vi "Configure Spurious Emission (Segment Sweep And Trace Setup).vi"(0 "VISA resource name":refnum<visa-resource-name>, 1 "Spurious Detection Mode":i32[](array[ring]) items=["Normal", "Positive", "Sample", "Negative", "RMS"], 5 "Spurious Mode (1:On)":i32(ring)=1 items=["Off", "On"], 7 "Spurious Auto Sweep Time":i32[](array[ring]) items=["Auto", "Manual"], 9 "Spurious Trace Point":i32[](array[ring]) items=["11", "21", "41", "51", "101", "201", "251", "401", "501", "1001", "2001", "5001", "10001"], 11 "error in (no error)":errorcluster, 12 "Spurious Storage Count":i32[](array[numeric]) min=2 max=9999, 13 "Spurious Sweep Time":dbl[](array[numeric]) min=0.001 max=1000.0) -> (4 "VISA resource name out":refnum<visa-resource-name>, 15 "error out":errorcluster)   [LabVIEW 2020, in "Anritsu Signal Analyzer Series.lvlib"]
doc: "Configures the sweep and trace for segment parameter of Spurious Emission measurement."
uses:
  Anritsu Signal Analyzer Series.lvlib
panel:
  # "s"
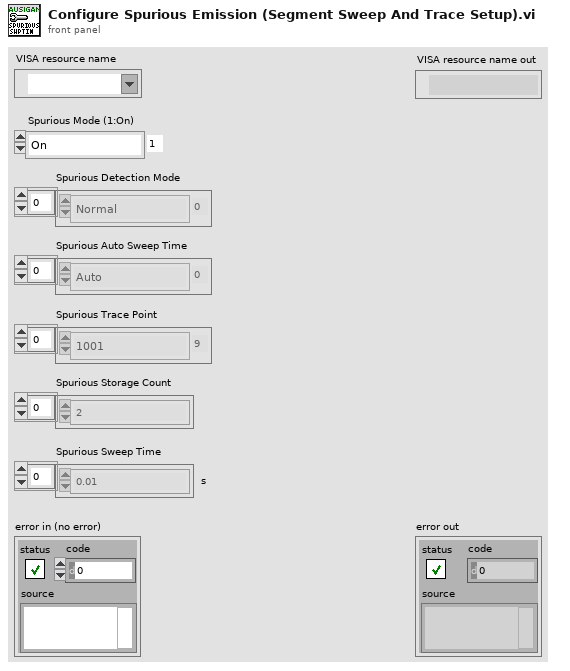
[diagram p1: front panel]
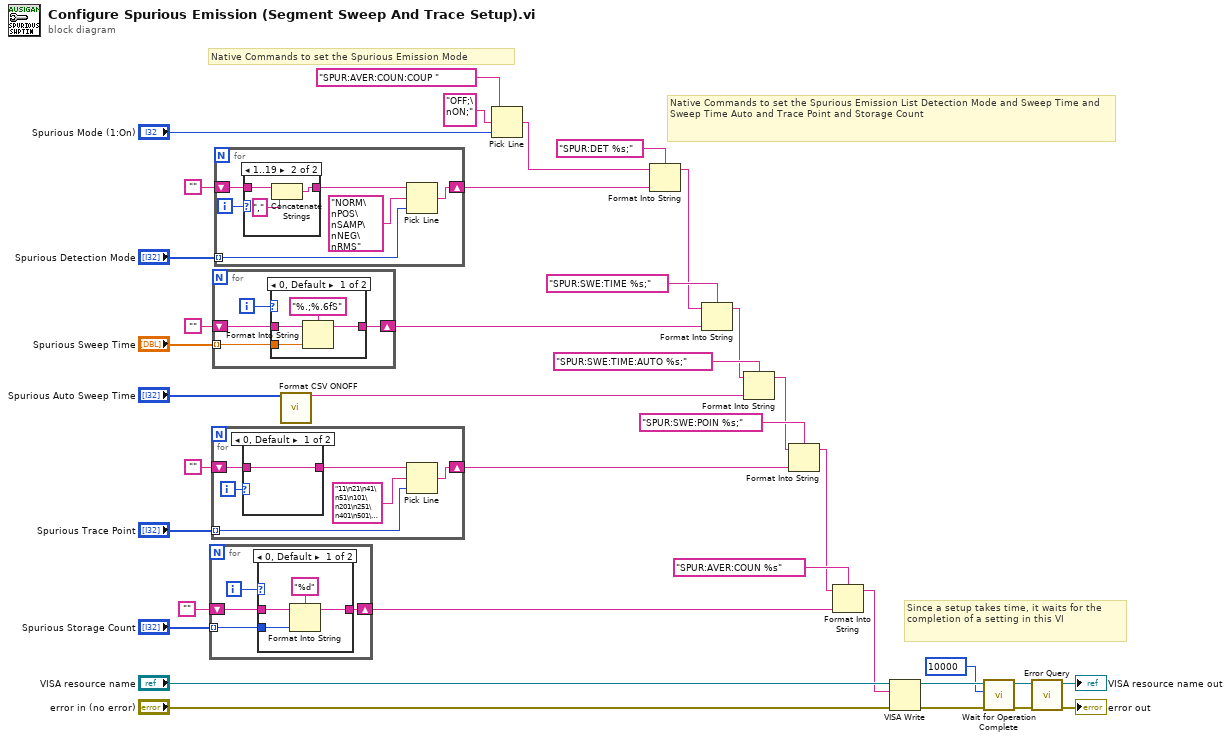
[diagram p0: block diagram]
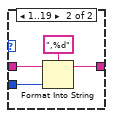
[diagram p2: hidden frame]
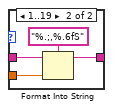
[diagram p3: hidden frame]
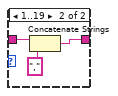
[diagram p4: hidden frame]
diagram:
  # "Since a setup takes time, it waits for the completion of a setting in this VI"
  # "Native Commands to set the Spurious Emission List Detection Mode and Sweep Time and Sweep Time Auto and Trace Point and Storage Count"
  # "Native Commands to set the Spurious Emission Mode"
  n1 = for {
    shift-right: [w38] -> w14
    shift-left: "" -> [w40]
    tunnel: "Spurious Storage Count" -> [w39] mode=indexing
    i -> [w41]
    n2 = case shown="0, Default" w41 {
      tunnel: w40 -> [w44 w47]
      tunnel: [w42 w46] -> w38
      tunnel: w39 -> [w43 w48]
      frame 0, Default {
        n3 = Format Into String(format string="%d" ("string"), initial string=w44, w43) -> (resulting string=w42:string)  [unwired: 1 in, 1 out]
      }
      frame 1..19 {
        n4 = Format Into String(format string=",%d" ("string"), initial string=w47, w48) -> (resulting string=w46:string)  [unwired: 1 in, 1 out]
      }
    }
  }
  n5 = for {
    shift-right: [w50] -> w22
    shift-left: "" -> [w54]
    tunnel: "Spurious Trace Point" -> [w51] mode=indexing
    i -> [w55]
    n6 = case shown="0, Default" w55 {
      tunnel: w54 -> [w56 w59]
      tunnel: [w56 w57] -> w52
      frame 0, Default {
      }
      frame 1..19 {
        n7 = Concatenate Strings(w59, "," ("string")) -> (w57:string)
      }
    }
    n8 = Pick Line(string ("")=w52, multi-line string="11\n21\n41\n51\n101\n201\n251\n401\n501\n1001\n2001\n5001\n10001" ("複数行文字列"), line index=w51) -> (output string=w50:string)
  }
  n9 = for {
    shift-right: [w60] -> w16
    shift-left: "" -> [w62]
    tunnel: "Spurious Sweep Time" -> [w61] mode=indexing
    i -> [w63]
    n10 = case shown="0, Default" w63 {
      tunnel: w62 -> [w66 w69]
      tunnel: [w64 w68] -> w60
      tunnel: w61 -> [w65 w70]
      frame 0, Default {
        n11 = Format Into String(format string="%.;%.6fS" ("string"), initial string=w66, w65) -> (resulting string=w64:string)  [unwired: 1 in, 1 out]
      }
      frame 1..19 {
        n12 = Format Into String(format string="%.;,%.6fS" ("string"), initial string=w69, w70) -> (resulting string=w68:string)  [unwired: 1 in, 1 out]
      }
    }
  }
  n13 = for {
    shift-right: [w73] -> w27
    shift-left: "" -> [w76]
    tunnel: "Spurious Detection Mode" -> [w72] mode=indexing
    i -> [w77]
    n14 = case shown="1..19" w77 {
      tunnel: w76 -> [w78 w81]
      tunnel: [w78 w79] -> w74
      frame 0, Default {
      }
      frame 1..19 {
        n15 = Concatenate Strings(w81, "," ("string")) -> (w79:string)
      }
    }
    n16 = Pick Line(string ("")=w74, multi-line string="NORM\nPOS\nSAMP\nNEG\nRMS" ("複数行文字列"), line index=w72) -> (output string=w73:string)
  }
  n17 = call "Format CSV ONOFF.vi"("Data_In"="Spurious Auto Sweep Time") -> ("Data_out"=w4:string)  [unwired: 14 in]
  n18 = Pick Line(string ("")="SPUR:AVER:COUN:COUP " ("_CommandSet"), multi-line string="OFF;\nON;" ("複数行文字列"), line index="Spurious Mode (1:On)") -> (output string=w8:string)
  n19 = Format Into String(format string="SPUR:DET %s;" ("_CommandSet"), initial string=w8, w27) -> (resulting string=w13:string)  [unwired: 1 in, 1 out]
  n20 = Format Into String(format string="SPUR:SWE:TIME %s;" ("_CommandSet"), initial string=w13, w16) -> (resulting string=w12:string)  [unwired: 1 in, 1 out]
  n21 = Format Into String(format string="SPUR:SWE:TIME:AUTO %s;" ("_CommandSet"), initial string=w12, w4) -> (resulting string=w11:string)  [unwired: 1 in, 1 out]
  n22 = Format Into String(format string="SPUR:SWE:POIN %s;" ("_CommandSet"), initial string=w11, w22) -> (resulting string=w19:string)  [unwired: 1 in, 1 out]
  n23 = Format Into String(format string="SPUR:AVER:COUN %s" ("_CommandSet"), initial string=w19, w14) -> (resulting string=w18:string)  [unwired: 1 in, 1 out]
  n24 = VISA Write(VISA resource name="VISA resource name", write buffer=w18, error in (no error)="error in (no error)") -> (VISA resource name out=w3:refnum<visa-resource-name>, error out=w2:errorcluster)  [unwired: 1 out]
  n25 = call "Wait for Operation Complete.vi"("error in (no error)"=w2, "Maximum Time (10000mSec)"=10000, "VISA resource name"=w3) -> ("error out"=w6:errorcluster, "VISA resource name out"=w7:refnum<visa-resource-name>)  [unwired: 7 in]
  n26 = call "Error Query.vi"("error in (no error)"=w6, "VISA resource name"=w7) -> ("error out"=→"error out":errorcluster, "VISA resource name out"=→"VISA resource name out":refnum<visa-resource-name>)  [unwired: 6 in, 2 out]
